vi "曲线判定demo.vi"() -> ()   [LabVIEW 2020]
panel:
  out "OK？":bool
  in  "Result":string[][](table)
  out "XY图":cluster{dbl[], dbl[]}[](graph)
  in  "文件路径输入控件":path
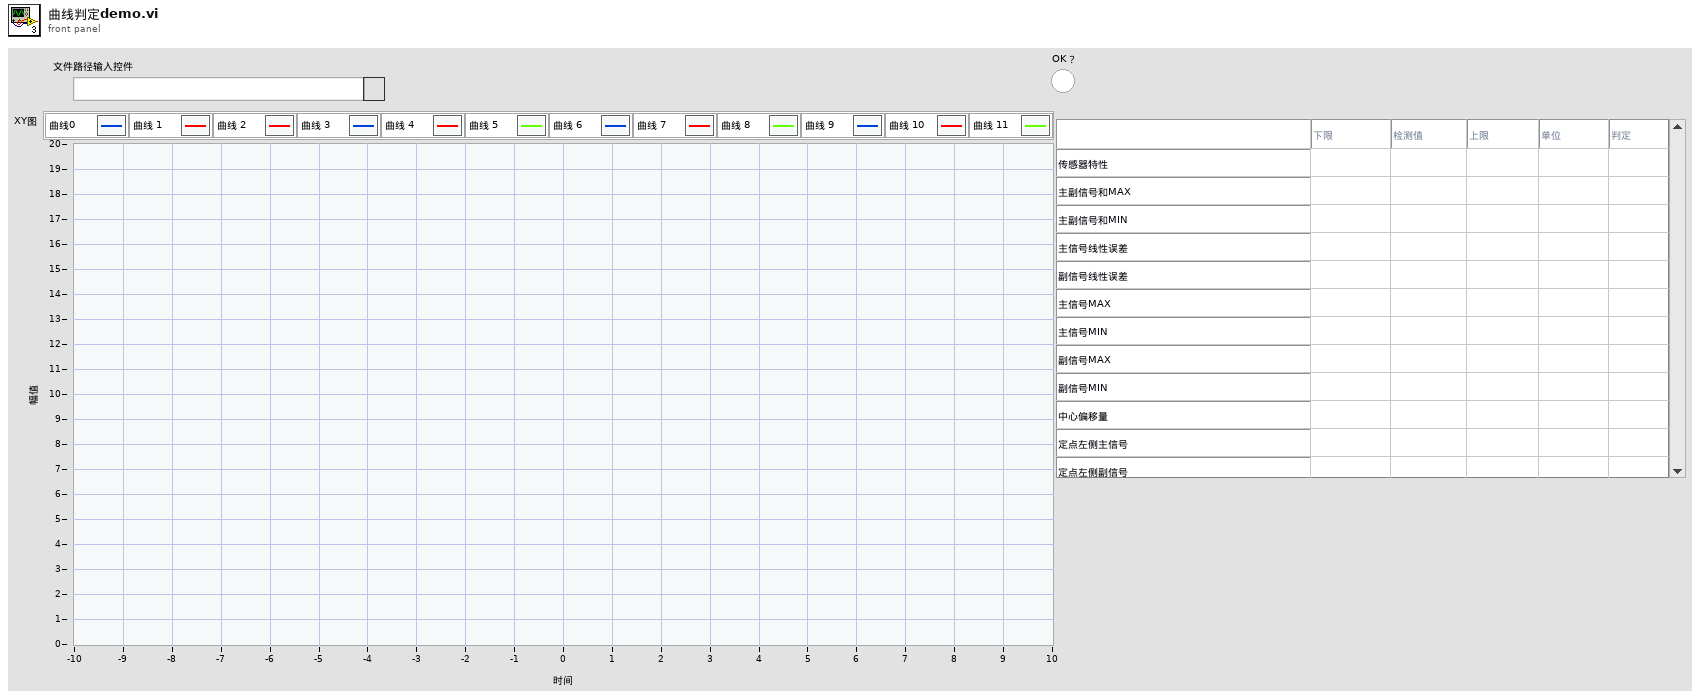
[diagram p1: front panel]
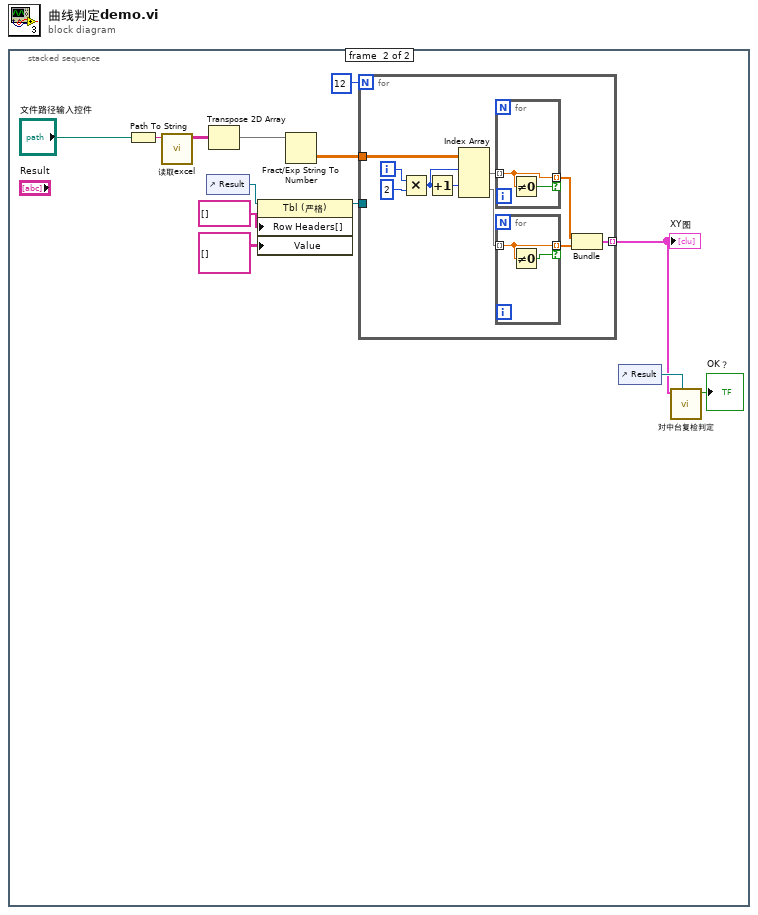
[diagram p0: block diagram]
diagram:
  n1 = stacked-sequence {
    frame #0 {
    }
    frame #1 {
      n2 = Path To String(path="文件路径输入控件") -> (string=w12:string)
      n3 = call "读取excel.vi"("Filename"=w12) -> ("数据"=w11:string[][])  [unwired: 10 in]
      n4 = control-ref of="Result"() -> (w2:refnum<vi>)
      n5 = Transpose 2D Array(2D array=w11) -> (transposed array=w10:string[][])
      n6 = property class="Tbl (严格)"(reference=w2, "Row Headers[]"=string[] [] ("行首字符串[]"), "Value"=string[][] [] ("值")) -> (reference out=w1:refnum<vi>)  [unwired: 1 in, 1 out]
      n7 = Fract/Exp String To Number(string=w10) -> (number=w9:dbl[][])  [unwired: 3 in, 1 out]
      n8 = for {
        N: 12 -> [_]
        tunnel: w9 -> [w23]
        tunnel: [w17] -> w6 mode=indexing
        tunnel: w1 -> [_]
        i -> [w21]
        n9 = Multiply(x=w21, y=2) -> (x*y=w16:i32)
        n10 = Increment(x=w16) -> (x+1=w15:i32)
        n11 = Index Array(array=w23, index (row) #1=w16, index (row) #2=w15) -> (element #1=w22:dbl[], element #2=w19:dbl[])  [unwired: 2 in]
        n12 = for {
          tunnel: w22 -> [w26] mode=indexing
          tunnel: [w26] -> w18 mode=indexing if=w27
          n13 = Not Equal To 0?(x=w26) -> (x != 0?=w27:bool)
        }
        n14 = for {
          tunnel: w19 -> [w24] mode=indexing
          tunnel: [w24] -> w14 mode=indexing if=w25
          n15 = Not Equal To 0?(x=w24) -> (x != 0?=w25:bool)
        }
        n16 = Bundle(w18, w14) -> (w17:cluster{dbl[], dbl[]})  [unwired: 1 in]
      }
      "XY图" <- w6
      n17 = control-ref of="Result"() -> (w7:refnum<vi>)
      n18 = call "对中台复检判定.vi"("Result"=w7, "XY曲线"=w6) -> ("OK？"=→"OK？":bool)  [unwired: 9 in]
    }
  }
